vi "P4CMD_Sup Path Array to Cmd Line String.vi"(6 "expand wildcards? (T)":bool=TRUE, 9 "modifiers":string[](array[string]), 11 "files":path[](array[path])) -> (1 "string output":string, 3 "converted file strings":string[](array[string]))   [LabVIEW 2017, in "NI_SCC_P4CMD.lvlib"]
uses:
  <vilib>/SourceControl/Providers/P4CMD/NI_SCC_P4CMD.lvlib
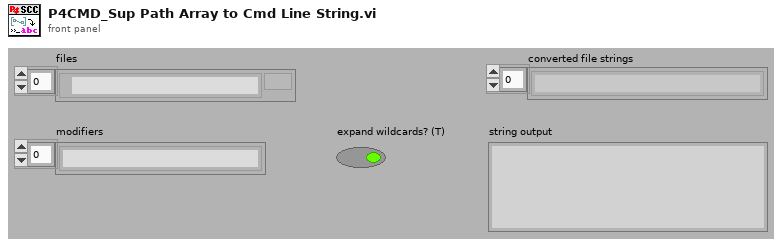
[diagram p1: front panel]
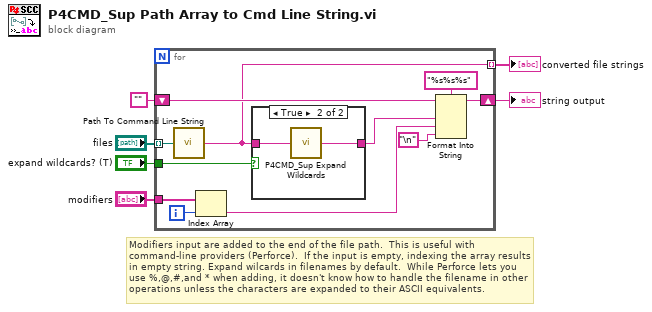
[diagram p0: block diagram]
diagram:
  # "Modifiers input are added to the end of the file path.  This is useful with command-line providers (Perforce).  If the input is empty, indexing the array results in empty string. Expand wilcards in filenames by default.  While Perforce lets you use %,@,#,and * when adding, it doesn't know how to handle the filename in other operations unless the characters are expanded to their ASCII equivalents."
  n1 = for {
    shift-right: [w16] -> w4
    shift-left: "" -> [w17]
    tunnel: "files" -> [w12] mode=indexing
    tunnel: "modifiers" -> [w15]
    tunnel: [w8] -> w2 mode=indexing
    tunnel: "expand wildcards? (T)" -> [w9]
    i -> [w14]
    n2 = call <vilib>:"Path To Command Line String.vi"("path"=w12) -> ("string"=w8:string)
    n3 = Index Array(array=w15, index=w14) -> (element=w13:string)
    n4 = case shown="True" w9 {
      tunnel: w8 -> [w18 w20]
      tunnel: [w18 w19] -> w7
      frame False {
        # "Check Out uses this VI to display list of files."
      }
      frame True {
        n5 = call <vilib>:"P4CMD_Sup Expand Wildcards.vi"("string input"=w20) -> ("string output"=w19:string)  [unwired: 4 in]
      }
    }
    n6 = Format Into String(format string="%s%s%s", initial string=w17, w7, w13, "\n") -> (resulting string=w16:string)  [unwired: 1 in, 1 out]
  }
  "string output" <- w4
  "converted file strings" <- w2
